vi "SphereSection.vi"(0 "Ducer":cluster{"radius":dbl, "theta":dbl, "phi":dbl} {"radius" format="%.2f"; "phi" format="%.2f"; "theta" format="%.2f"}, 2 "Rotate":dbl format="%.2f", 3 "P":cluster{"x":dbl, "y":dbl, "z":dbl}={"x"=-4.0, "y"=0.0, "z"=4.0} {"x" format="%.2f"; "z" format="%.2f"; "y" format="%.2f"}) -> (1 "thetas":dbl[](array[numeric]) format="%.2f", 4 "phis":dbl[](array[numeric]) format="%.2f", 6 "x matrix":dbl[][](array[numeric]) format="%.2f", 7 "y matrix":dbl[][](array[numeric]) format="%.2f", 8 "z matrix":dbl[][](array[numeric]) format="%.2f")   [LabVIEW 2022 SP3]
uses:
  <vilib>/Analysis/NI_AALPro.lvlib
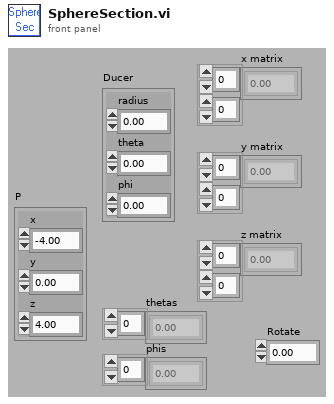
[diagram p1: front panel]
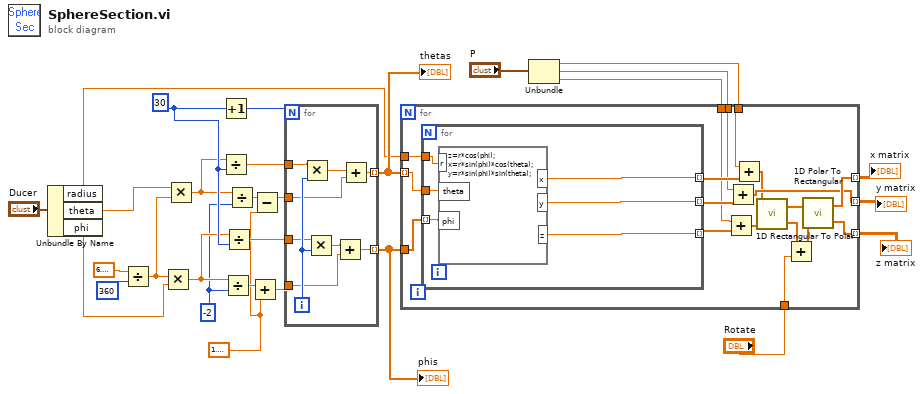
[diagram p0: block diagram]
diagram:
  w28 = 30
  w15 = -2
  w12 = 1.5707963267948966
  n1 = Unbundle By Name("Ducer") -> ("radius"=w8:dbl, "theta"=w7:dbl, "phi"=w6:dbl)
  n2 = Divide(x=6.283185307179586, y=360) -> (x/y=w25:dbl)
  n3 = Multiply(x=w25, y=w6) -> (x*y=w23:dbl)
  n4 = Multiply(x=w7, y=w25) -> (x*y=w24:dbl)
  n5 = Increment(x=w28) -> (x+1=w29:i32)
  n6 = Divide(x=w24, y=w28) -> (x/y=w16:dbl)
  n7 = Divide(x=w23, y=w15) -> (x/y=w26:dbl)
  n8 = Divide(x=w23, y=w28) -> (x/y=w17:dbl)
  n9 = Divide(x=w24, y=w15) -> (x/y=w11:dbl)
  n10 = Add(x=w26, y=w12) -> (x+y=w27:dbl)
  n11 = Subtract(x=w11, y=w12) -> (x-y=w10:dbl)
  n12 = for {
    N: w29 -> [_]
    tunnel: w27 -> [w32]
    tunnel: w10 -> [w30]
    tunnel: w16 -> [w37]
    tunnel: w17 -> [w36]
    tunnel: [w35] -> w18 mode=indexing
    tunnel: [w34] -> w19 mode=indexing
    i -> [w38]
    n13 = Multiply(x=w37, y=w38) -> (x*y=w33:dbl)
    n14 = Multiply(x=w36, y=w38) -> (x*y=w31:dbl)
    n15 = Add(x=w31, y=w32) -> (x+y=w34:dbl)
    n16 = Add(x=w33, y=w30) -> (x+y=w35:dbl)
  }
  "thetas" <- w18
  "phis" <- w19
  n17 = Unbundle("P") -> ("x"=w4:dbl, "y"=w3:dbl, "z"=w2:dbl)
  n18 = for {
    tunnel: w18 -> [w55] mode=indexing
    tunnel: w19 -> [w54]
    tunnel: w8 -> [w56]
    tunnel: [w48] -> w20 mode=indexing
    tunnel: [w45] -> w21 mode=indexing
    tunnel: [w50] -> w22 mode=indexing
    tunnel: "Rotate" -> [w51]
    tunnel: w4 -> [w42]
    tunnel: w3 -> [w41]
    tunnel: w2 -> [w40]
    n19 = for {
      tunnel: w56 -> [w62]
      tunnel: w55 -> [w61]
      tunnel: w54 -> [w60] mode=indexing
      tunnel: [w59] -> w47 mode=indexing
      tunnel: [w58] -> w46 mode=indexing
      tunnel: [w57] -> w44 mode=indexing
      n20 = formula code="z=r*cos(phi);\nx=r*sin(phi)*cos(theta);\ny=r*sin(phi)*sin(theta);"("r"=w62, "phi"=w60, "theta"=w61) -> ("x"=w59:dbl, "y"=w58:dbl, "z"=w57:dbl)
    }
    n21 = Add(x=w40, y=w44) -> (x+y=w43:dbl[])
    n22 = Add(x=w41, y=w46) -> (x+y=w45:dbl[])
    n23 = Add(x=w42, y=w47) -> (x+y=w39:dbl[])
    n24 = call <vilib>:"1D Rectangular To Polar.vi"("X"=w39, "Y"=w43) -> ("Magnitude"=w49:dbl[], "Phase"=w53:dbl[])  [unwired: 1 out]
    n25 = Add(x=w53, y=w51) -> (x+y=w52:dbl[])
    n26 = call <vilib>:"1D Polar To Rectangular.vi"("Magnitude"=w49, "Phase"=w52) -> ("X"=w48:dbl[], "Y"=w50:dbl[])  [unwired: 1 out]
  }
  "z matrix" <- w22
  "y matrix" <- w21
  "x matrix" <- w20
